vi "Get Wheel Parameter by Name as String.vi"(8 "error in (no error)":errorcluster, 10 "parameter name":string, 11 "wheel in":refnum<class "NI_Robotics_Mecanum Wheel.lvclass">) -> (0 "error out":errorcluster, 1 "found?":bool, 2 "parameter value":string, 3 "wheel out":refnum<class "NI_Robotics_Mecanum Wheel.lvclass">)   [LabVIEW 2017, in "NI_Robotics_Mecanum Wheel.lvclass"]
uses:
  <vilib>/robotics/Steering/Mecanum Wheel/NI_Robotics_Mecanum Wheel.lvclass
  <vilib>/robotics/Steering/Mecanum Wheel/NI_Robotics_Mecanum Wheel.lvclass/NI_Robotics_Mecanum Wheel.ctl
  <vilib>/robotics/Steering/Wheel/NI_Robotics_Wheel.lvclass
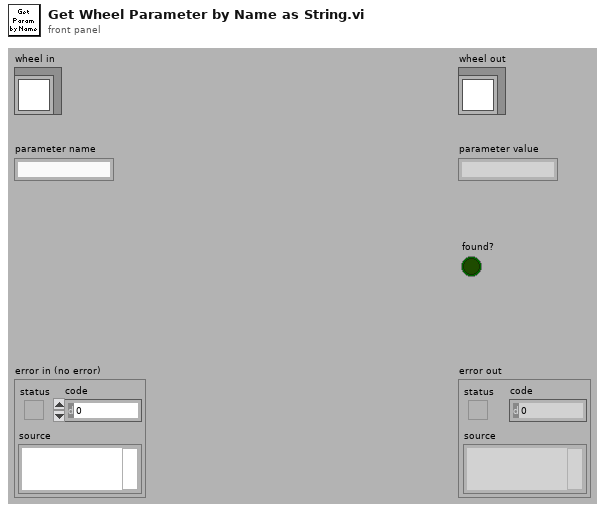
[diagram p1: front panel]
types:
  T1 = typedef "NI_Robotics_Mecanum Wheel.lvclass/Roller Orientation.ctl" = u16
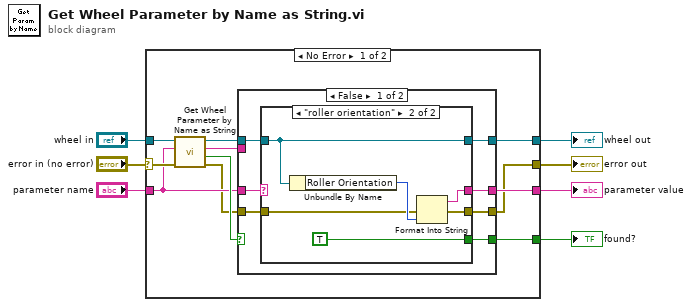
[diagram p0: block diagram]
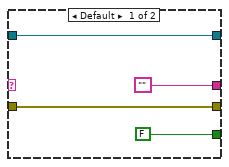
[diagram p2: hidden frame]
diagram:
  n1 = case shown="No Error" "error in (no error)" {
    selector: "error in (no error)" -> [w17 w40]
    tunnel: [w8 w40] -> w5
    tunnel: [w15 _] -> w3
    tunnel: [w13 _] -> w4
    tunnel: [w11 w41] -> w6
    tunnel: "parameter name" -> [w10 _]
    tunnel: "wheel in" -> [w18 w41]
    frame No Error {
      n2 = call-parent "Get Wheel Parameter by Name as String.vi"("error in (no error)"=w17, "parameter name"=w10, "wheel in"=w18) -> ("error out"=w9:errorcluster, "found?"=w16:bool, "parameter value"=w14:string, "wheel out"=w12:refnum<class "NI_Robotics_Mecanum Wheel.lvclass">)  [unwired: 5 in]
      n3 = case shown="False" w16 {
        selector: w16 -> [_ w39]
        tunnel: [w22 w39] -> w15
        tunnel: w14 -> [_ w38]
        tunnel: [w21 w38] -> w13
        tunnel: w12 -> [w25 w37]
        tunnel: [w23 w37] -> w11
        tunnel: w10 -> [w24 _]
        tunnel: w9 -> [w20 w36]
        tunnel: [w19 w36] -> w8
        frame False {
          n4 = case shown="\"roller orientation\"" w24 {
            tunnel: w25 -> [w29 w35]
            tunnel: [w29 w35] -> w23
            tunnel: [FALSE TRUE] -> w22
            tunnel: ["" ("parameter value") w32] -> w21
            tunnel: w20 -> [w26 w31]
            tunnel: [w26 w30] -> w19
            frame Default {
            }
            frame "roller orientation" {
              n5 = Unbundle By Name(w35) -> ("Roller Orientation"=w33:T1)
              n6 = Format Into String(error in=w31, w33) -> (resulting string=w32:string, error out=w30:errorcluster)  [unwired: 2 in]
            }
          }
        }
        frame True {
        }
      }
    }
    frame Error {
    }
  }
  "error out" <- w5
  "wheel out" <- w6
  "found?" <- w3
  "parameter value" <- w4
